vi "34401 - Read meas.vi"(2 "error in (no error)":errorcluster, 3 "address string":string) -> (0 "error out":errorcluster, 1 "number":dbl)   [LabVIEW 2014]
doc: "This VI will read whatever measurement has been selected from the measurement config or math config VI's. This includes dB, dBm, null, and limit.\n\nThe VI will wait up to the timeout value for data to become available. If the time expires prior to reading the data, you will receive a timeout error. The meaning of \"timeout\" is dependent upon the interface used and number of points collected. See below for details.\n\nGPIB\ninternal buffer (<512 points) -- RQS is asserted only after all data is collected and generally\n requires more time than VISA Read. Thus timeout is essentially the time needed for all\n data to be collected and RQS assented (VISA RQS timeout). \n\noutput buffer -- RQS is asserted after the first trigger point and then the driver waits on the\n meter to transmit data. Thus timeout is essentially the time needed for all data to be\n transmitted (VISA Read timeout).\n\n\nSerial (Not GPIB)\ninternal buffer (<512 points) -- Data transmission only begins after all data is collected and\n generally requires more time than VISA Read.\n\noutput buffer -- Data transmission begins immediately.\n\nIn both cases, the driver continually polls (ASRL Avail Num) the seral buffer and then reads only the data present. Although less efficient than performing a single VISA Read, this method significantly reduces processor overhead and frees system resources. Timeout is calculated using the tick count and is the time required for data collection and transmission. The VISA Read uses the default timeout value specified in HP34401A Initialize.vi. A VISA Read timeout is highly unlikely since data is being read from the seral buffer and not from the meter."
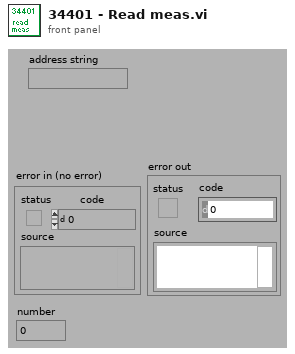
[diagram p1: front panel]
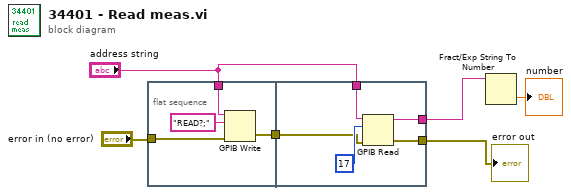
[diagram p0: block diagram]
diagram:
  n1 = flat-sequence {
    tunnel: "address string" -> [w9]
    tunnel: "error in (no error)" -> [w8]
    tunnel: [w7] -> w4
    tunnel: "address string" -> [w14]
    tunnel: w4 -> [w13]
    tunnel: [w12] -> w3
    tunnel: [w11] -> w2
    frame #0 {
      n2 = GPIB Write(0:w9, 1:"READ?;" ("data"), 3:w8) -> (6:w7:errorcluster)  [unwired: 2 in, 1 out]
    }
    frame #1 {
      n3 = GPIB Read(0:w14, 1:17 ("byte count"), 3:w13) -> (5:w11:string, 7:w12:errorcluster)  [unwired: 2 in, 1 out]
    }
  }
  n4 = Fract/Exp String To Number(string=w2) -> (number=→"number":dbl)  [unwired: 3 in, 1 out]
  "error out" <- w3
